vi "HGF_DIMCommand.appendData2Variant.vi"(0 "initData":variant, 2 "typeDescriptor":string, 5 "error in (no error)":errorcluster) -> (14 "dup initData":variant, 19 "error out":errorcluster)   [LabVIEW 2012, in "HGF_DIM.lvlib" / "HGF_DIMCommand.lvclass"]
uses:
  HGF_DIMCommand.lvclass
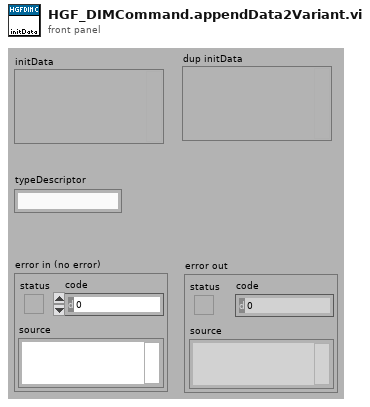
[diagram p1: front panel]
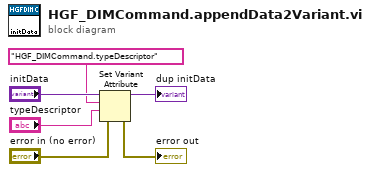
[diagram p0: block diagram]
diagram:
  n1 = Set Variant Attribute(Variant="initData", name="HGF_DIMCommand.typeDescriptor", value="typeDescriptor", error in="error in (no error)") -> (Variant out=→"dup initData":variant, error out=→"error out":errorcluster)  [unwired: 1 out]
